vi "TMP007 Read.vi"(8 "error in (no error)":errorcluster, 9 "Thermopile Setting":T1 {"Last Temp Readings"."Ambient Temp (°F)" format="%.2f °F"; "Last Temp Readings"."Ambient Temp (°C)" format="%.2f °C"; "Last Temp Readings"."Object Temp (°F)" format="%.2f °F"; "Last Temp Readings"."Object Temp (°C)" format="%.2f °C"; "Samples to Average" items=["1 sample, .26s conversion"=0, "2 samples, .51s conversion"=512, "4 samples, 1.01s conversion"=1024, "8 samples, 2.01s conversion"=1536, "16 samples, 4.01s conversion"=2048]; "I2C Slave Address" format="%.0x"}, 11 "LINX Resource in":T3) -> (0 "error out":errorcluster, 1 "Thermopile Status":T1 {"Last Temp Readings"."Ambient Temp (°F)" format="%.2f °F"; "Last Temp Readings"."Ambient Temp (°C)" format="%.2f °C"; "Last Temp Readings"."Object Temp (°F)" format="%.2f °F"; "Last Temp Readings"."Object Temp (°C)" format="%.2f °C"; "Samples to Average" items=["1 sample, .26s conversion"=0, "2 samples, .51s conversion"=512, "4 samples, 1.01s conversion"=1024, "8 samples, 2.01s conversion"=1536, "16 samples, 4.01s conversion"=2048]; "I2C Slave Address" format="%.0x"}, 2 "Temp Readings":T2 {"Ambient Temp (°F)" format="%.2f °F"; "Ambient Temp (°C)" format="%.2f °C"; "Object Temp (°F)" format="%.2f °F"; "Object Temp (°C)" format="%.2f °C"}, 3 "LINX Resource":T3, 4 "Conversion Time (ms)":dbl)   [LabVIEW 2017]
uses:
  <vilib>/MakerHub/LINX/Private/Type Defs/LINX Ref.ctl
  <vilib>/MakerHub/LINX/Private/Type Defs/Platform.ctl
  <vilib>/MakerHub/LINX/Private/Type Defs/Interface.ctl
  <vilib>/MakerHub/LINX/Private/Device/Type Defs/LINX Device Config.ctl
  <vilib>/MakerHub/LINX/Private/Device/Type Defs/TCP Config.ctl
  <vilib>/MakerHub/LINX/Private/Device/Type Defs/Channels.ctl
  Type Defs/tempReadings.ctl
  Type Defs/thermopileSettings.ctl
  <vilib>/MakerHub/LINX/LMH-LINX.lvlib
  <vilib>/MakerHub/LINX/Private/Device/Device.lvlib
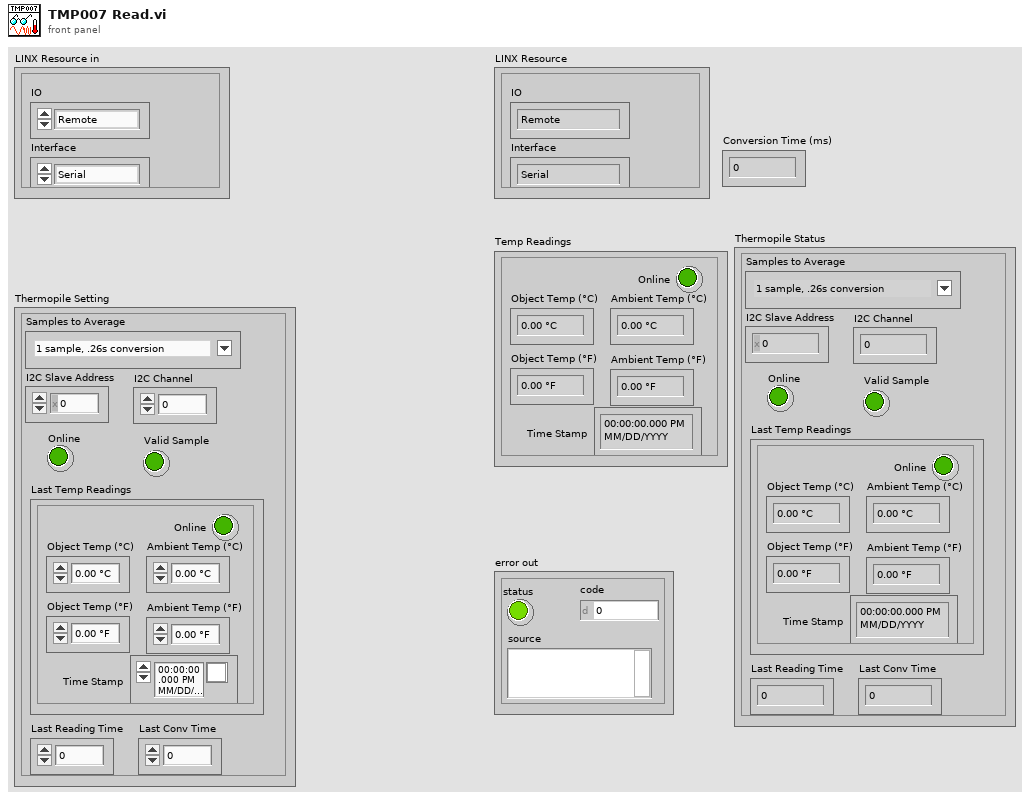
[diagram p1: front panel]
types:
  T1 = typedef "thermopileSettings.ctl" = cluster{"Online":bool, "I2C Channel":u8, "I2C Slave Address":u8, "Valid Sample":bool, "Samples to Average":u16, "Last Temp Readings":T2, "Last Reading Time":dbl, "Last Conv Time":dbl}
  T2 = typedef "tempReadings.ctl" = cluster{"Object Temp (°C)":dbl, "Object Temp (°F)":dbl, "Ambient Temp (°C)":dbl, "Ambient Temp (°F)":dbl, "Online":bool, "Time Stamp":timestamp}
  T3 = typedef "LMH-LINX.lvlib/LINX Ref.ctl" = cluster{"IO":T4, "Interface":T5, "LINX Device Config":T6}
  T4 = typedef "LMH-LINX.lvlib/Platform.ctl" = enum16{"Remote", "Local"}
  T5 = typedef "LMH-LINX.lvlib/Interface.ctl" = enum16{"Serial", "TCP"}
  T6 = typedef "LMH-LINX.lvlib/Device.lvlib/LINX Device Config.ctl" = cluster{"Interface":T5, "COM Port":refnum<visa-resource-name>, "TCP Configuration":T7, "Device Family":u8, "Device ID":u8, "Device Name":string, "TCP Ref":refnum<k5>, "Channels":T8}
  T7 = typedef "LMH-LINX.lvlib/Device.lvlib/TCP Config.ctl" = cluster{"IP Address":string, "Port":u16}
  T8 = typedef "LMH-LINX.lvlib/Channels.ctl" = cluster{"DI":u8[], "DO":u8[], "AI":u8[], "AO":u8[], "PWM":u8[], "QE":u8[], "UART":u8[], "I2C 2":u8[], "SPI":u8[], "CAN":u8[], "Servo":u8[], "AI Ref (V)":dbl, "AI Resolution (Bits)":u8, "AO Ref (V)":dbl, "AO Resolution (Bits)":u8}
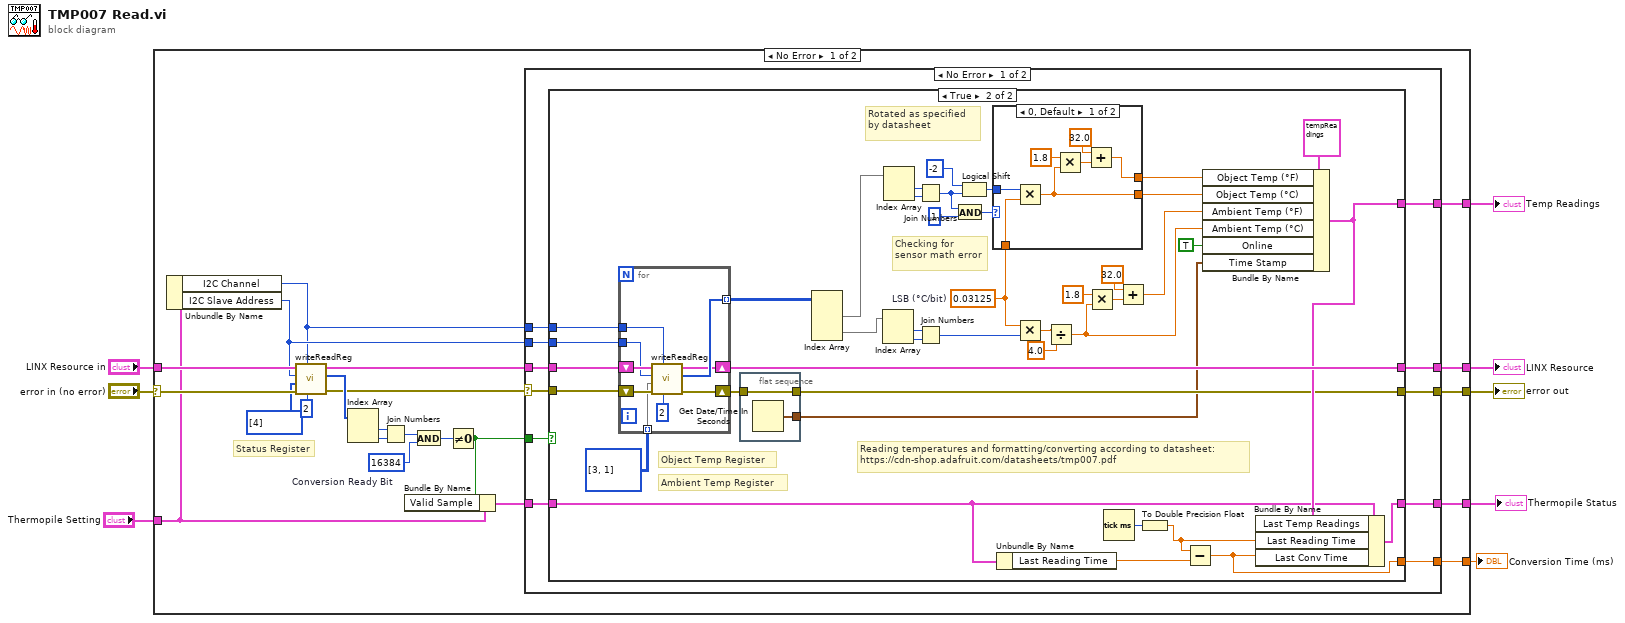
[diagram p0: block diagram]
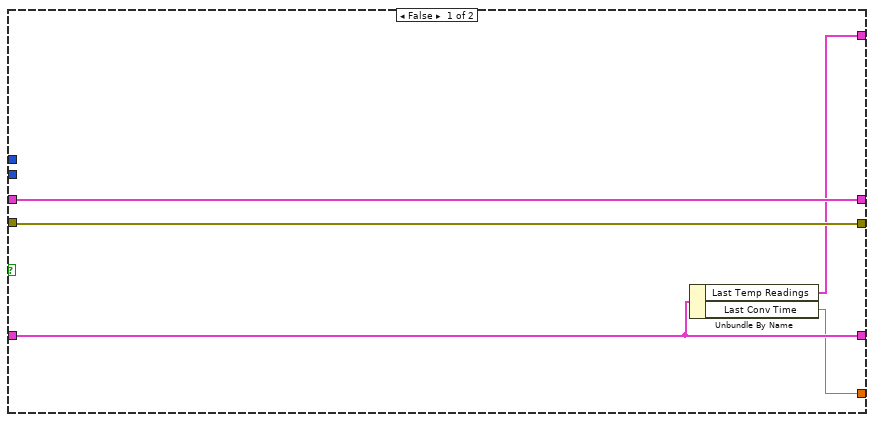
[diagram p2: hidden frame]
diagram:
  n1 = case shown="No Error" "error in (no error)" {
    selector: "error in (no error)" -> [w25 w108]
    tunnel: [w30 w109] -> w8
    tunnel: [w29 w108] -> w7
    tunnel: [w28 _] -> w6
    tunnel: "LINX Resource in" -> [w27 w109]
    tunnel: "Thermopile Setting" -> [w13 w107]
    tunnel: [w15 w107] -> w2
    tunnel: [w10 _] -> w1
    frame No Error {
      w20 = u16 16384  # Conversion Ready Bit
      # "Status Register"
      n2 = Unbundle By Name(w13) -> ("I2C Channel"=w11:u8, "I2C Slave Address"=w12:u8)
      n3 = call "writeReadReg.vi"("Bytes To Read"=u8 2, "I2C Channel"=w11, "error in"=w25, "Data"=u8[] [4], "I2C Slave Address"=w12, "LINX Resource in"=w27) -> ("error out"=w9:errorcluster, "Bytes Read"=w17:u8[], "LINX Resource out"=w26:T3)  [unwired: 3 in]
      n4 = Index Array(array=w17) -> (element #1=w23:u8, element #2=w22:u8)  [unwired: 2 in]
      n5 = Join Numbers(hi=w23, lo=w22) -> ((hi.lo)=w21:u16)
      n6 = And(x=w21, y=w20) -> (x .and. y?=w19:u16)
      n7 = Not Equal To 0?(x=w19) -> (x != 0?=w16:bool)
      n8 = Bundle By Name(cluster=w13, "Valid Sample"=w16) -> (w14:T1)
      n9 = case shown="No Error" w9 {
        selector: w9 -> [w31 _]
        tunnel: [w41 w106] -> w30
        tunnel: [w40 _] -> w29
        tunnel: [w39 _] -> w28
        tunnel: w26 -> [w38 w106]
        tunnel: w16 -> [w37 _]
        tunnel: [w36 _] -> w15
        tunnel: w14 -> [w35 _]
        tunnel: w12 -> [w34 _]
        tunnel: w11 -> [w33 _]
        tunnel: [w32 _] -> w10
        frame No Error {
          n10 = case shown="True" w37 {
            tunnel: [w46 w87] -> w41
            tunnel: [w45 w48] -> w40
            tunnel: [w43 w58] -> w39
            tunnel: w31 -> [w45 w65]
            tunnel: w38 -> [w46 w64]
            tunnel: w33 -> [_ w63]
            tunnel: w34 -> [_ w62]
            tunnel: [w44 w57] -> w36
            tunnel: w35 -> [w44 w56]
            tunnel: [w42 w52] -> w32
            frame False {
              n11 = Unbundle By Name(w44) -> ("Last Temp Readings"=w43:T2, "Last Conv Time"=w42:dbl)
            }
            frame True {
              w73 = 0.03125  # LSB (°C/bit)
              # "Reading temperatures and formatting/converting according to datasheet:\nhttps://cdn-shop.adafruit.com/datasheets/tmp007.pdf"
              # "Rotated as specified by datasheet"
              # "Checking for sensor math error"
              # "Ambient Temp Register"
              # "Object Temp Register"
              n12 = for {
                tunnel: w62 -> [w103]
                tunnel: w63 -> [w102]
                shift-right: [w97] -> w49
                shift-left: w65 -> [w105]
                shift-right: [w98] -> w87
                shift-left: w64 -> [w104]
                tunnel: u8[][] [[3], [1]] ("Data") -> [w101] mode=indexing
                tunnel: [w99] -> w85 mode=indexing
                n13 = call "writeReadReg.vi"("Bytes To Read"=u8 2, "I2C Channel"=w102, "error in"=w105, "Data"=w101, "I2C Slave Address"=w103, "LINX Resource in"=w104) -> ("error out"=w97:errorcluster, "Bytes Read"=w99:u8[], "LINX Resource out"=w98:T3)  [unwired: 3 in]
              }
              n14 = flat-sequence {
                tunnel: w49 -> [w89]
                tunnel: [w89] -> w48
                tunnel: [w88] -> w47
                frame #0 {
                  n15 = Get Date/Time In Seconds() -> (seconds since 1Jan1904=w88:timestamp)
                }
              }
              n16 = Index Array(array=w85) -> (element #1=w84:u8[], element #2=w83:u8[])  [unwired: 4 in]
              n17 = Index Array(array=w83) -> (element #1=w80:u8, element #2=w79:u8)  [unwired: 2 in]
              n18 = Index Array(array=w84) -> (element #1=w81:u8, element #2=w82:u8)  [unwired: 2 in]
              n19 = Join Numbers(hi=w81, lo=w82) -> ((hi.lo)=w77:u16)
              n20 = Join Numbers(hi=w80, lo=w79) -> ((hi.lo)=w75:u16)
              n21 = And(x=w77, y=u16 1) -> (x .and. y?=w72:u16)
              n22 = Logical Shift(y=i16 -2, x=w77) -> (x << y=w74:u16)
              n23 = case shown="0, Default" w72 {
                tunnel: w74 -> [w96 _]
                tunnel: w73 -> [w95 _]
                tunnel: [w91 _] -> w71
                tunnel: [w90 _] -> w70
                frame 0, Default {
                  n24 = Multiply(x=w96, y=w95) -> (x*y=w91:dbl)
                  n25 = Multiply(x=1.8, y=w91) -> (x*y=w92:dbl)
                  n26 = Add(x=32.0, y=w92) -> (x+y=w90:dbl)
                }
                frame 1 {
                  # "Sensor math error found on sensor"
                }
              }
              n27 = Unbundle By Name(w56) -> ("Last Reading Time"=w54:dbl)
              n28 = Multiply(x=w73, y=w75) -> (x*y=w61:dbl)
              n29 = Divide(x=w61, y=4.0) -> (x/y=w60:dbl)
              n30 = Multiply(x=1.8, y=w60) -> (x*y=w69:dbl)
              n31 = Tick Count (ms)() -> (millisecond timer value=w55:u32)
              n32 = Add(x=32.0, y=w69) -> (x+y=w66:dbl)
              n33 = To Double Precision Float(number=w55) -> (double precision float=w53:dbl)
              n34 = Subtract(x=w53, y=w54) -> (x-y=w52:dbl)
              n35 = Bundle By Name(cluster=T2 {"Object Temp (°C)"=0.0, "Object Temp (°F)"=0.0, "Ambient Temp (°C)"=0.0, "Ambient Temp (°F)"=0.0, "Online"=FALSE, "Time Stamp"=timestamp(0 s since 1904-01-01)} ("Temp Readings"), "Object Temp (°F)"=w70, "Object Temp (°C)"=w71, "Ambient Temp (°F)"=w66, "Ambient Temp (°C)"=w60, "Online"=TRUE, "Time Stamp"=w47) -> (w58:T2)
              n36 = Bundle By Name(cluster=w56, "Last Temp Readings"=w58, "Last Reading Time"=w53, "Last Conv Time"=w52) -> (w57:T1)
            }
          }
        }
        frame Error {
        }
      }
    }
    frame Error {
    }
  }
  "error out" <- w7
  "LINX Resource" <- w8
  "Temp Readings" <- w6
  "Thermopile Status" <- w2
  "Conversion Time (ms)" <- w1
